vi "Unpack Message Identifier.vi"(10 "packed message identifier":u32) -> (2 "message identifiers":cluster{"Port":u8, "Label":u8, "SDI":u8})   [LabVIEW 2020]
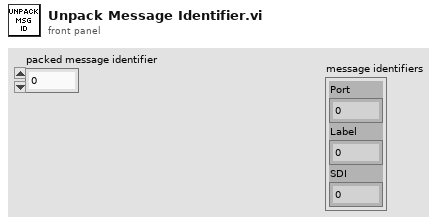
[diagram p1: front panel]
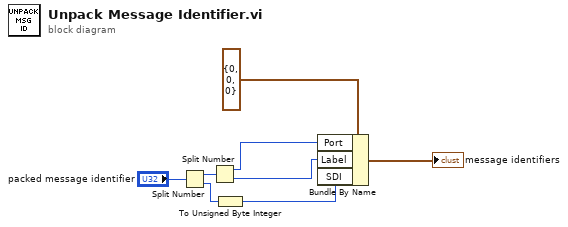
[diagram p0: block diagram]
diagram:
  n1 = Split Number(x="packed message identifier") -> (hi(x)=w5:u16, lo(x)=w2:u16)
  n2 = Split Number(x=w5) -> (hi(x)=w4:u8, lo(x)=w3:u8)
  n3 = To Unsigned Byte Integer(number=w2) -> (unsigned 8bit integer=w1:u8)
  n4 = Bundle By Name(cluster=cluster{"Port":u8, "Label":u8, "SDI":u8} {"Port"=0, "Label"=0, "SDI"=0} ("message identifiers"), "Port"=w4, "Label"=w3, "SDI"=w1) -> (→"message identifiers":cluster{"Port":u8, "Label":u8, "SDI":u8})
